vi "AutoIncreasePath.vi"(3 "Error In":errorcluster, 5 "TDMS file path":path=path "C:/code/2010-10-14 cat experiment/2010_10_14_file_01.tdms") -> (0 "Error Out":errorcluster, 2 "TDMS file path out":path)   [LabVIEW 2011]
uses:
  <vilib>/regexp/Match Regular Expression.xnode
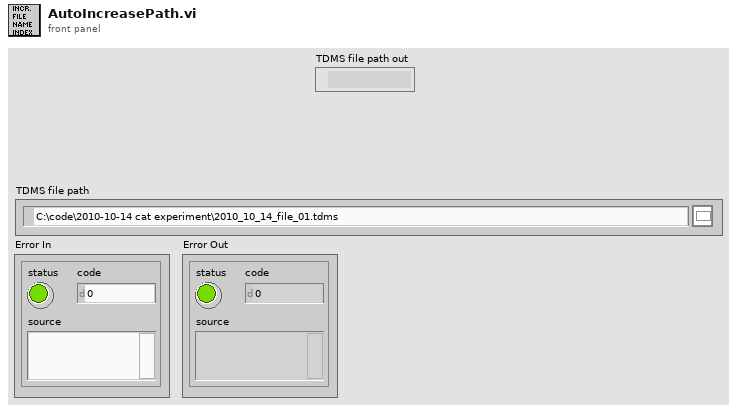
[diagram p1: front panel]
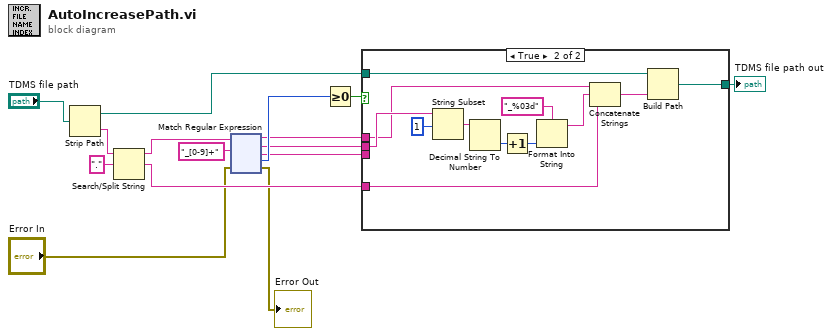
[diagram p0: block diagram]
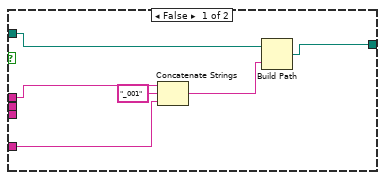
[diagram p2: hidden frame]
diagram:
  n1 = Strip Path(path="TDMS file path") -> (stripped path=w8:path, name=w6:string)
  n2 = Search/Split String(string=w6, search string/char (-)=".") -> (substring before match=w4:string, match + rest of string=w3:string)  [unwired: 1 in, 1 out]
  n3 = xnode "Match Regular Expression"("input string"=w4, "regular expression"="_[0-9]+", "error in"="Error In") -> ("before match"=w11:string, "whole match"=w10:string, "after match"=w9:string, "offset past match"=w12:i32, "error out"=→"Error Out":errorcluster)  [unwired: 3 in]
  n4 = Greater Or Equal To 0?(x=w12) -> (x >= 0?=w13:bool)
  n5 = case shown="True" w13 {
    tunnel: w11 -> [w19 w25]
    tunnel: w10 -> [_ w28]
    tunnel: w9 -> [_ _]
    tunnel: w8 -> [w21 w26]
    tunnel: [w20 w23] -> w7
    tunnel: w3 -> [w17 w22]
    frame False {
      n6 = Concatenate Strings(w19, "_001" ("string"), w17) -> (w16:string)
      n7 = Build Path(base path=w21, name or relative path=w16) -> (appended path=w20:path)
    }
    frame True {
      n8 = String Subset(string=w28, offset (0)=1) -> (substring=w29:string)  [unwired: 1 in]
      n9 = Decimal String To Number(string=w29) -> (number=w30:i32)  [unwired: 2 in, 1 out]
      n10 = Increment(x=w30) -> (x+1=w31:i32)
      n11 = Format Into String(format string="_%03d", w31) -> (resulting string=w24:string)  [unwired: 2 in, 1 out]
      n12 = Concatenate Strings(w25, w24, w22) -> (w33:string)
      n13 = Build Path(base path=w26, name or relative path=w33) -> (appended path=w23:path)
    }
  }
  "TDMS file path out" <- w7
